vi "Configure AC Line Trigger Slope [AT] Core.vi"(8 "error in (no error)":errorcluster, 10 "ac line trigger slope (Positive)":i32(ring)=1 items=["Positive"=1, "Negative"=2, "Either"=3], 11 "IVI_Scope in":refnum<class "IVI_Scope.lvclass">) -> (0 "error out":errorcluster, 3 "IVI_Scope out":refnum<class "IVI_Scope.lvclass">)   [LabVIEW 2013, in "IVI_Scope.lvlib" / "IVI_Scope.lvclass"]
doc: "This VI configures the slope of the AC Line trigger.\n\nNote (1) This VI affects instrument behavior only if the trigger type is IVISCOPE_VAL_AC_LINE_TRIGGER. Call the IviScope Configure Trigger VI to set the trigger type before calling this VI.\n(2) This VI is part of the IviScopeAcLineTrigger [AT] extension group."
uses:
  IVI_Scope.lvclass
  IVI_Scope.lvclass/IVI_Scope.ctl
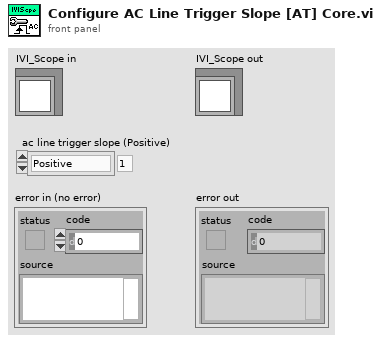
[diagram p1: front panel]
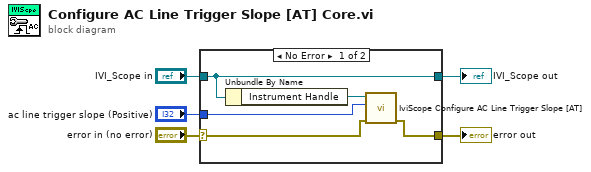
[diagram p0: block diagram]
diagram:
  n1 = case shown="No Error" "error in (no error)" {
    selector: "error in (no error)" -> [w10 w12]
    tunnel: [w9 w12] -> w4
    tunnel: [w8 w11] -> w2
    tunnel: "IVI_Scope in" -> [w8 w11]
    tunnel: "ac line trigger slope (Positive)" -> [w6 _]
    frame No Error {
      n2 = Unbundle By Name(w8) -> ("Instrument Handle"=w7:refnum<k15>)
      n3 = call <vilib>:"IviScope Configure AC Line Trigger Slope [AT].vi"("error in (no error)"=w10, "ac line trigger slope (Positive)"=w6, "instrument handle"=w7) -> ("error out"=w9:errorcluster)  [unwired: 7 in, 1 out]
    }
    frame Error {
    }
  }
  "error out" <- w4
  "IVI_Scope out" <- w2
